vi "1.vi"(8 "error in (no error)":errorcluster, 10 "pattern":string="LabVIEW *", 11 "dup path":path) -> (0 "error in (no error) (dup)":errorcluster, 1 "file names":string[](array[string]), 2 "folder names":string[](array[string]), 3 "dup path (dup)":path)   [LabVIEW 2014]
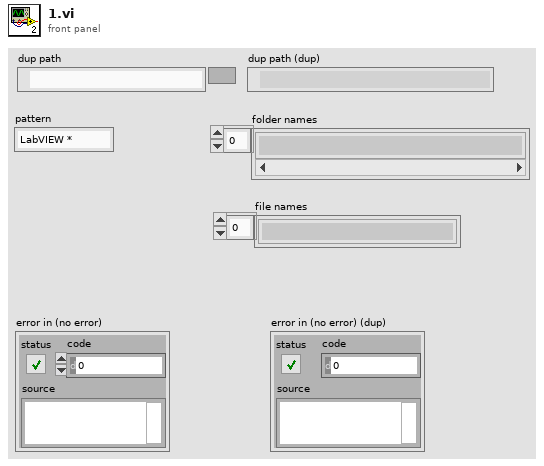
[diagram p1: front panel]
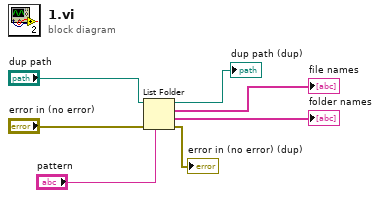
[diagram p0: block diagram]
diagram:
  n1 = List Folder(path="dup path", pattern="pattern", error in="error in (no error)") -> (path out=→"dup path (dup)":path, filenames=→"file names":string[], folder names=→"folder names":string[], error out=→"error in (no error) (dup)":errorcluster)  [unwired: 1 in]
